vi "Drive Train Motion Track File.vi"(4 "Use Ave":bool, 6 "Ka":dbl, 7 "Kv":dbl, 9 "Auton Step":T2, 10 "PID Settings":T1, 11 "file (use dialog)":path) -> (0 "error out":errorcluster, 3 "json error":errorcluster)   [LabVIEW 2015]
uses:
  Support/LightningPID Settings.ctl
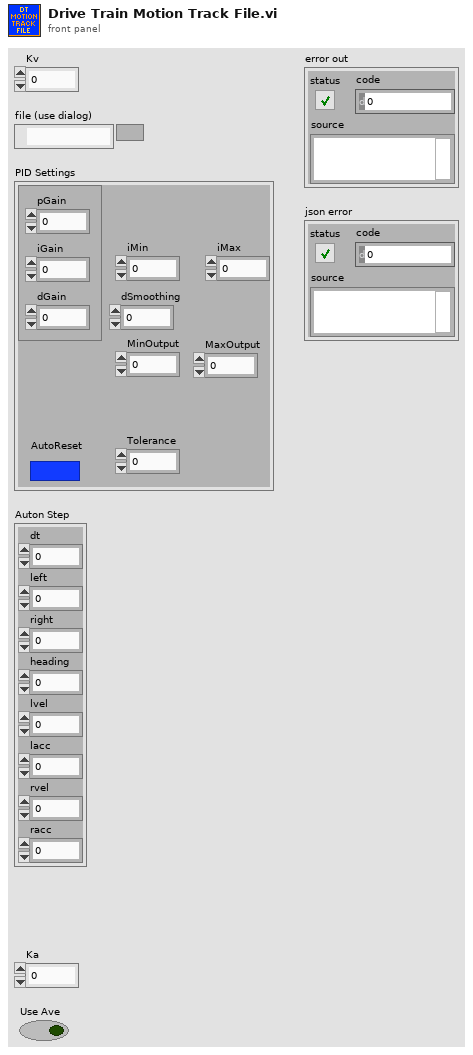
[diagram p1: front panel]
types:
  T1 = typedef "LightningPID Settings.ctl" = cluster{"iMax":dbl, "iMin":dbl, "iGain":dbl, "pGain":dbl, "dGain":dbl, "MaxOutput":dbl, "MinOutput":dbl, "AutoReset":bool, "Tolerance":dbl, "dSmoothing":dbl}
  T2 = cluster{"dt":dbl, "left":dbl, "right":dbl, "heading":dbl, "lvel":dbl, "lacc":dbl, "rvel":dbl, "racc":dbl}
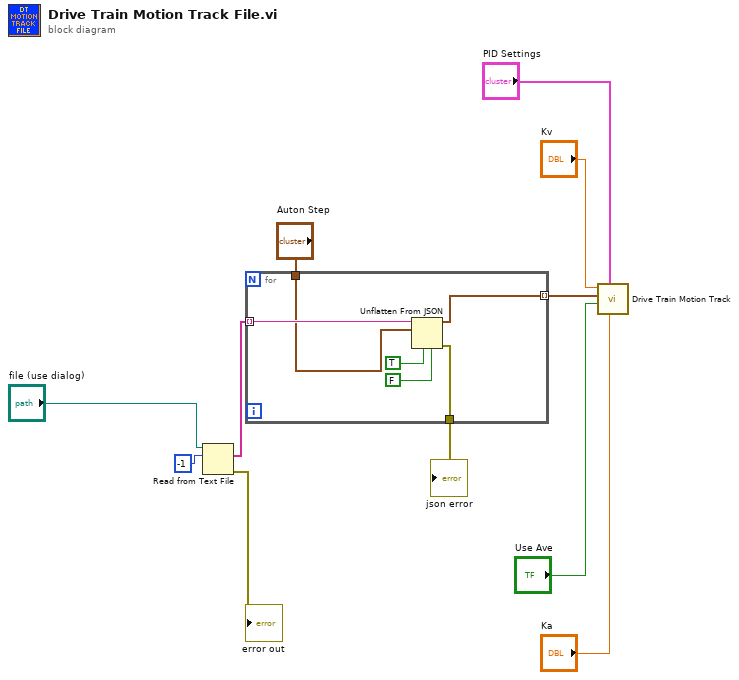
[diagram p0: block diagram]
diagram:
  n1 = Read from Text File(file (use dialog)="file (use dialog)", count=-1) -> (text=w4:string[], error out=→"error out":errorcluster)  [unwired: 2 in, 2 out]
  n2 = for {
    tunnel: w4 -> [w17] mode=indexing
    tunnel: [w16] -> w5 mode=indexing
    tunnel: "Auton Step" -> [w13]
    tunnel: [w12] -> w11
    n3 = Unflatten From JSON(JSON string=w17, type and defaults=w13, default null elements? (F)=TRUE, strict validation? (F)=FALSE) -> (value=w16:T2, error out=w12:errorcluster)  [unwired: 3 in]
  }
  "json error" <- w11
  n4 = call "Drive Train Motion Track.vi"("Ka"="Ka", "PID Settings"="PID Settings", "Use Ave"="Use Ave", "Array"=w5, "Kv"="Kv") -> ()  [unwired: 7 in]
